vi "x-axis.vi"(8 "error in (no error)":errorcluster, 11 "Wavelength iHR320 in":refnum<class "Wavelength ActiveX.lvclass">) -> (0 "error out":errorcluster, 1 "Label":string, 2 "Unit":string, 3 "Wavelength iHR320 out":refnum<class "Wavelength ActiveX.lvclass">)   [LabVIEW 2015, in "Wavelength ActiveX.lvclass"]
uses:
  Wavelength ActiveX.lvclass
  Scanner/Scanner.lvclass
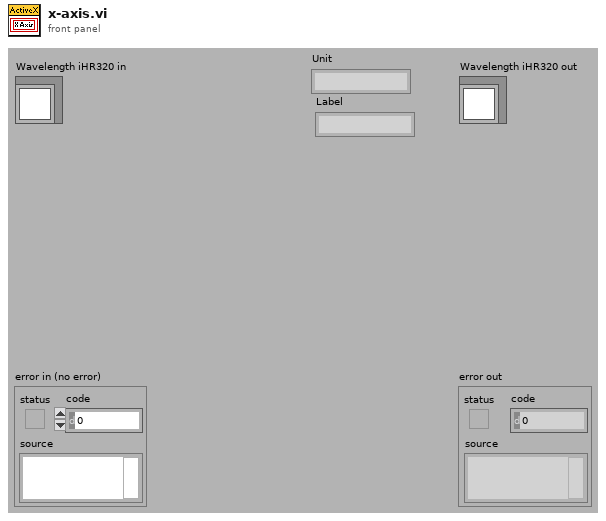
[diagram p1: front panel]
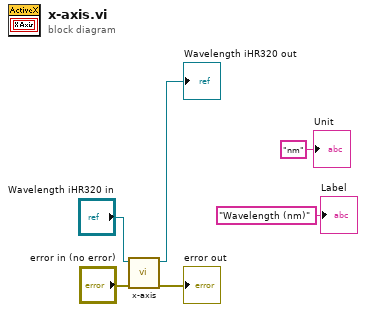
[diagram p0: block diagram]
diagram:
  n1 = call-parent "x-axis.vi"("error in (no error)"="error in (no error)", "Scanner in"="Wavelength iHR320 in") -> ("error out"=→"error out":errorcluster, "Scanner out"=→"Wavelength iHR320 out":refnum<class "Wavelength ActiveX.lvclass">)  [unwired: 6 in, 2 out]
  "Label" <- "Wavelength (nm)" ("Label")
  "Unit" <- "nm" ("Unit")
